vi "20220114_01.vi"() -> ()   [LabVIEW 2019]
panel:
  in  "執行程式":bool
  in  "置中前面板":bool
  in  "關閉前面板":bool
  in  "打開前面板":bool
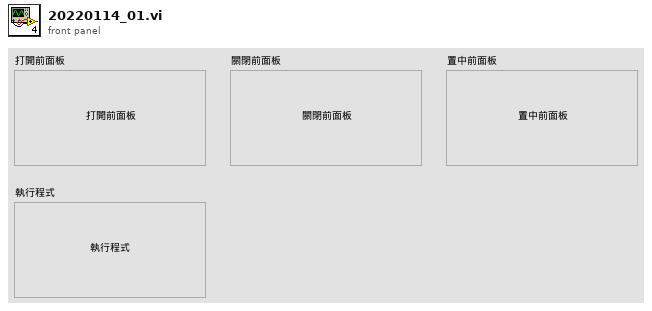
[diagram p1: front panel]
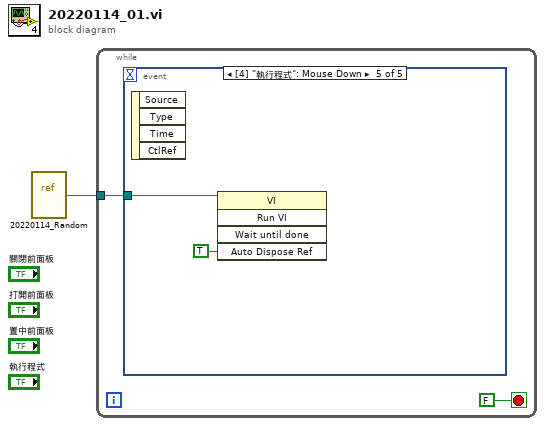
[diagram p0: block diagram]
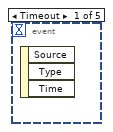
[diagram p2: hidden frame]
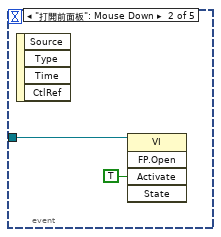
[diagram p3: hidden frame]
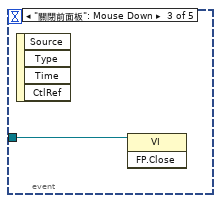
[diagram p4: hidden frame]
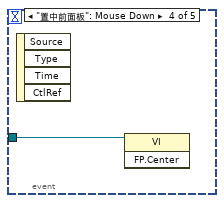
[diagram p5: hidden frame]
diagram:
  n1 = vi-ref "20220114_Random.vi"() -> (w1:refnum<vi>)
  n2 = while {
    tunnel: w1 -> [w3]
    stop <- FALSE stop-if-true
    n3 = event shown="[4] \"執行程式\": Mouse Down" {
      selector: _ -> [_ _ _ _ _]
      dyn-events: _ -> [_ _ _ _ _]
      timeout: _ -> [_ _ _ _ _]
      tunnel: w3 -> [_ w5 w6 w7 w9]
      event Timeout {
        n4 = event-data() -> ()  [unwired: 1 in, 3 out]
      }
      event "打開前面板": Mouse Down {
        n5 = event-data() -> ()  [unwired: 1 in, 4 out]
        n6 = invoke class="VI" method="FP.Open"(reference=w5, "Activate"=TRUE ("Activate?")) -> ()  [unwired: 3 in, 5 out]
      }
      event "關閉前面板": Mouse Down {
        n7 = event-data() -> ()  [unwired: 1 in, 4 out]
        n8 = invoke class="VI" method="FP.Close"(reference=w6) -> ()  [unwired: 2 in, 3 out]
      }
      event "置中前面板": Mouse Down {
        n9 = event-data() -> ()  [unwired: 1 in, 4 out]
        n10 = invoke class="VI" method="FP.Center"(reference=w7) -> ()  [unwired: 2 in, 3 out]
      }
      event "執行程式": Mouse Down {
        n11 = event-data() -> ()  [unwired: 1 in, 4 out]
        n12 = invoke class="VI" method="Run VI"(reference=w9, "Auto Dispose Ref"=TRUE ("Auto Dispose Reference")) -> ()  [unwired: 3 in, 5 out]
      }
    }
  }
